vi "view.vi"() -> ()   [LabVIEW 2022 SP3]
uses:
  <vilib>/Utility/file.llb/Read Delimited Spreadsheet (string).vi
panel:
  out "Image 2":T1(plugin-control)
  in  "File Path 2":path
  out "子数组 2":string[](array[string])
  in  "索引 (行)":i32
  out "all rows 2":string[][](array[string]) caption="所有行"
  out "元素 4":string
  out "元素 3":string
  out "元素 2":string
  out "元素":string
  out "子数组":string[][](array[string])
  out "all rows":string[][](array[string]) caption="所有行"
  in  "File Path":path
  in  "Save File Path":path
  out "Image":T1(plugin-control)
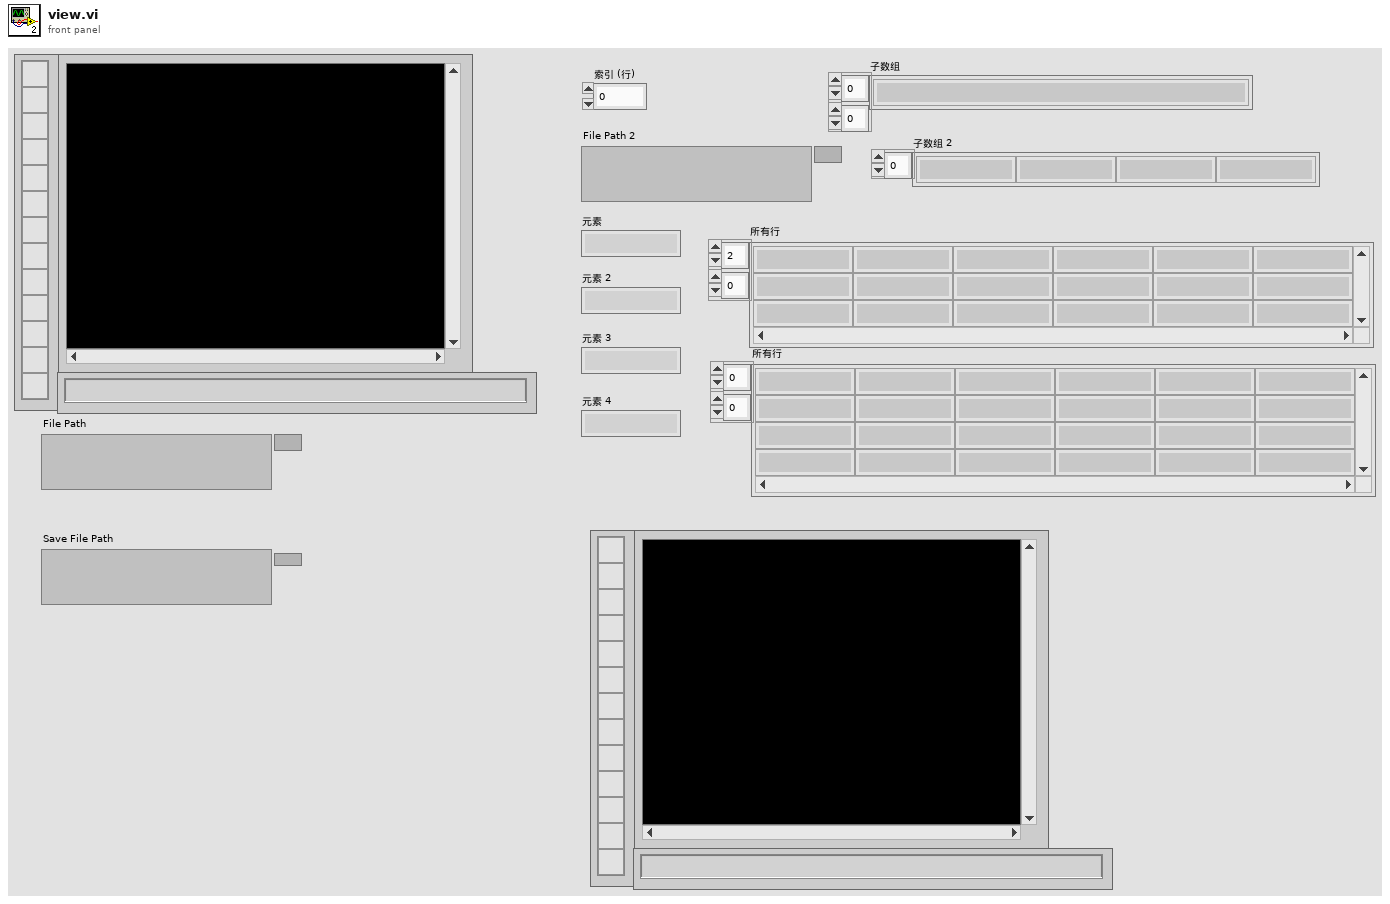
[diagram p1: front panel]
types:
  T1 = typedef "IMAQ Image.ctl" = refnum<image>
  T2 = typedef "Image Type" = u32
  T3 = typedef "IMAQ Rectangle" = cluster{"Left":i32, "Top":i32, "Right":i32, "Bottom":i32, "Rotation":dbl}
  T4 = enum16{"open", "replace", "create", "open or create", "replace or create", "replace or create with confirmation"}
  T5 = cluster{"Desired Font (Application)":enum16{"User-specified Font", "Application Font", "System Font", "Dialog Font"}, "[User-specified Font]":cluster{"Font Name":string, "Size":i16, "Strikeout?":bool, "Italic?":bool, "Underline?":bool, "Outline?":bool, "Shadow?":bool, "Bold?":bool, "Rotation Angle":dbl}, "Horizontal Alignment":i16, "Vertical Alignment":i16}
  T6 = cluster{"Global Rectangle":i32[], "Contours":cluster{"Contour Type":u32, "ROI Type":u32, "Points":i32[]}[]}
  T7 = cluster{"Contour Type":u32, "ROI Type":u32, "Points":i32[]}[]
  T8 = cluster{"Contour Type":u32, "ROI Type":u32, "Points":i32[]}
  T9 = typedef "ROI Descriptor" = cluster{"Global Rectangle":i32[], "Contours":cluster{"ID":enum32{"External", "Internal"}, "Type":u32, "Coordinates":i32[]}[]}
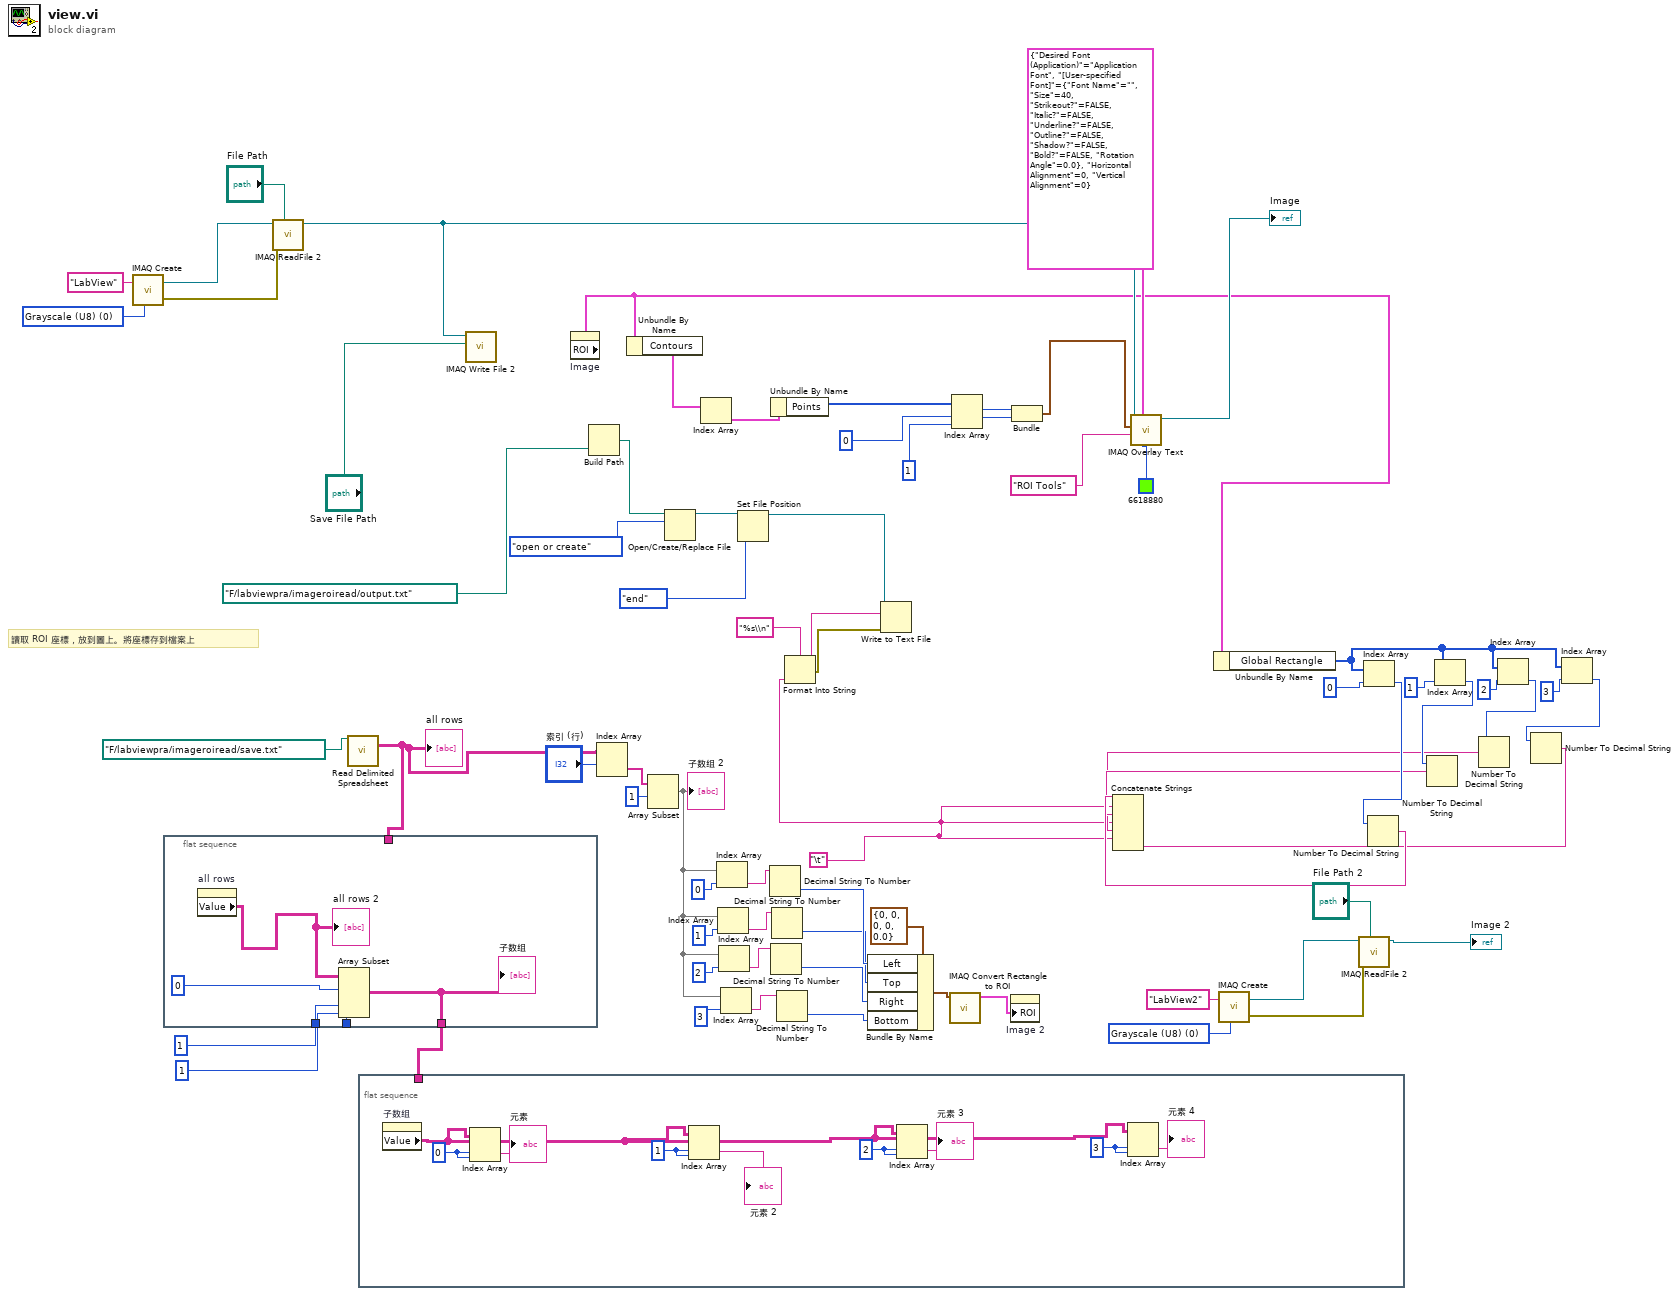
[diagram p0: block diagram]
diagram:
  w6 = T2 0 items=["Grayscale (U8)", "Grayscale (I16)", "Grayscale (SGL)", "Complex (CSG)", "RGB (U32)", "HSL (U32)", "RGB (U64)", "Grayscale (U16)"] ("Image Type")
  w28 = "\t"
  w71 = T2 0 items=["Grayscale (U8)", "Grayscale (I16)", "Grayscale (SGL)", "Complex (CSG)", "RGB (U32)", "HSL (U32)", "RGB (U64)", "Grayscale (U16)"] ("Image Type")
  # "讀取 ROI 座標，放到圖上。將座標存到檔案上"
  n1 = call "IMAQ Create"("Image Name"="LabView", "Image Type"=w71) -> ("New Image"=w74:T1, "error out"=w73:errorcluster)  [unwired: 3 in]
  n2 = flat-sequence {
    tunnel: 1 -> [w79]
    tunnel: 1 -> [w78]
    tunnel: w26 -> [_]
    tunnel: [w75] -> w27
    frame #0 {
      n3 = property on="all rows" class="Arr (严格)"() -> ("Value"=w76:string[][])  [unwired: 2 in, 2 out]
      "all rows 2" <- w76
      n4 = Array Subset(array=w76, index (row)=0, index (col)=w78, length (col)=w79) -> (w75:string[][])  [unwired: 1 in]
      "子数组" <- w75
    }
  }
  n5 = call "IMAQ ReadFile 2"("File Path"="File Path", "error in (no error)"=w73, "Image"=w74) -> ("Image Out"=w59:T1)  [unwired: 4 in, 4 out]
  n6 = call-poly <vilib>:"Read Delimited Spreadsheet.vi"("file path (dialog if empty)"=path "F:/labviewpra/imageroiread/save.txt" ("中间文件位置")) -> ("all rows"=w26:string[][])  [unwired: 9 in, 5 out]
  "all rows" <- w26
  n7 = flat-sequence {
    tunnel: w27 -> [_]
    frame #0 {
      w84 = 3
      w85 = 2
      w86 = 1
      w88 = 0
      n8 = property on="子数组" class="Arr (严格)"() -> ("Value"=w83:string[][])  [unwired: 2 in, 2 out]
      n9 = Index Array(array=w83, index (row)=w88, index (col)=w88) -> (element=→"元素":string)
      n10 = Index Array(array=w83, index (row)=w86, index (col)=w86) -> (element=→"元素 2":string)
      n11 = Index Array(array=w83, index (row)=w85, index (col)=w85) -> (element=→"元素 3":string)
      n12 = Index Array(array=w83, index (row)=w84, index (col)=w84) -> (element=→"元素 4":string)
    }
  }
  n13 = call-poly "IMAQ Write File 2"("File Path"="Save File Path", "Image"=w59) -> ()  [unwired: 8 in, 2 out]
  n14 = property on="Image" class="ImageControl"() -> ("ROI"=w37:T6)  [unwired: 2 in, 2 out]
  n15 = Build Path(name or relative path=path "F:/labviewpra/imageroiread/output.txt" ("名称或相对路径")) -> (appended path=w54:path)  [unwired: 1 in]
  n16 = Index Array(array=w26, index (row)="索引 (行)") -> (element=w24:string[])  [unwired: 1 in]
  n17 = Unbundle By Name(w37) -> ("Contours"=w68:T7)
  n18 = Array Subset(array=w24, index=1 ("索引")) -> (w22:string[])  [unwired: 1 in]
  "子数组 2" <- w22
  n19 = Open/Create/Replace File(file path (use dialog)=w54, operation (0:open)=T4."open or create" ("操作(0:open)")) -> (refnum out=w52:refnum<file>)  [unwired: 4 in, 2 out]
  n20 = Index Array(array=w68) -> (element=w67:T8)  [unwired: 1 in]
  n21 = Index Array(array=w22, index=0) -> (element=w17:string)
  n22 = Index Array(array=w22, index=1) -> (element=w14:string)
  n23 = Index Array(array=w22, index=2) -> (element=w16:string)
  n24 = Index Array(array=w22, index=3) -> (element=w15:string)
  n25 = Set File Position(refnum=w52, from (0:start)=enum16{"start", "end", "current"}."end" ("自（0:起始）")) -> (refnum out=w50:refnum<file>)  [unwired: 2 in, 1 out]
  n26 = Decimal String To Number(string=w17) -> (number=w11:i32)  [unwired: 2 in, 1 out]
  n27 = Unbundle By Name(w67) -> ("Points"=w66:i32[])
  n28 = Decimal String To Number(string=w16) -> (number=w9:i32)  [unwired: 2 in, 1 out]
  n29 = Decimal String To Number(string=w14) -> (number=w10:i32)  [unwired: 2 in, 1 out]
  n30 = Decimal String To Number(string=w15) -> (number=w8:i32)  [unwired: 2 in, 1 out]
  n31 = Bundle By Name(cluster=T3 {"Left"=0, "Top"=0, "Right"=0, "Bottom"=0, "Rotation"=0.0} ("Rectangle"), "Left"=w11, "Top"=w10, "Right"=w9, "Bottom"=w8) -> (w13:T3)
  n32 = call "IMAQ Convert Rectangle to ROI"("Rectangle"=w13) -> ("ROI Descriptor"=w1:T9)  [unwired: 8 in, 1 out]
  n33 = Index Array(array=w66, index #1=0 ("索引"), index #2=1 ("索引")) -> (element #1=w63:i32, element #2=w62:i32)
  n34 = property on="Image 2" class="ImageControl"("ROI"=w1) -> ()  [unwired: 2 in, 2 out]
  n35 = Bundle(w63, w62) -> (w61:cluster{i32, i32})  [unwired: 1 in]
  n36 = call "IMAQ Overlay Text"("Text Color (black)"=u32 6618880, "Font, Size & Style"=T5 {"Desired Font (Application)"=enum."Application Font", "[User-specified Font]"={"Font Name"="", "Size"=40, "Strikeout?"=FALSE, "Italic?"=FALSE, "Underline?"=FALSE, "Outline?"=FALSE, "Shadow?"=FALSE, "Bold?"=FALSE, "Rotation Angle"=0.0}, "Horizontal Alignment"=0, "Vertical Alignment"=0}, "String"="ROI Tools", "Origin"=w61, "Image"=w59) -> ("Image Out"=→"Image":T1)  [unwired: 5 in, 1 out]
  n37 = Unbundle By Name(w37) -> ("Global Rectangle"=w39:i32[])
  n38 = call "IMAQ Create"("Image Name"="LabView2", "Image Type"=w6) -> ("New Image"=w3:T1, "error out"=w4:errorcluster)  [unwired: 3 in]
  n39 = call "IMAQ ReadFile 2"("File Path"="File Path 2", "error in (no error)"=w4, "Image"=w3) -> ("Image Out"=→"Image 2":T1)  [unwired: 4 in, 4 out]
  n40 = Index Array(array=w39, index=0) -> (element=w43:i32)
  n41 = Number To Decimal String(number=w43) -> (decimal integer string=w36:string)  [unwired: 1 in]
  n42 = Index Array(array=w39, index=1) -> (element=w42:i32)
  n43 = Number To Decimal String(number=w42) -> (decimal integer string=w35:string)  [unwired: 1 in]
  n44 = Index Array(array=w39, index=2) -> (element=w41:i32)
  n45 = Number To Decimal String(number=w41) -> (decimal integer string=w34:string)  [unwired: 1 in]
  n46 = Index Array(array=w39, index=3) -> (element=w40:i32)
  n47 = Number To Decimal String(number=w40) -> (decimal integer string=w33:string)  [unwired: 1 in]
  n48 = Concatenate Strings(w36, w28, w35, w28, w34, w28, w33) -> (w32:string)
  n49 = Format Into String(format string="%s\\n" ("格式字符串"), w32) -> (resulting string=w49:string, error out=w38:errorcluster)  [unwired: 2 in]
  n50 = Write to Text File(file (use dialog)=w50, text=w49, error in=w38) -> ()  [unwired: 1 in, 3 out]
